vi "Read_Write_Calibrations.vi"(6 "Silent?":bool, 7 "Task":enum16{"Save", "Read", "List"}(ring)=enum."Read", 9 "Calibration name":string="Default", 11 "Settings in":T1={"Name of test"="", "Date"=timestamp(0 s since 1904-01-01), "Location"="", "Template"="", "Soundcard"="", "resolution"=32, "Sampling rate"=48000, "Ch1 Gain "=25.0, "Ch2 Gain"=10.0, "Sample time (s)"=0.3, "Pre-trigger (s)"=0.01, "Hammer Threshold"=10.0, "Positions"=12, "Taps/Position"=5, "Set Names"="", "Freq resolution"=10.0, "Hammer cutoff"=0.0, "Mic cutoff"=0.0, "Double bounce "=0.0, "Hammer Cal"=10.0, "dB Offset"=0.0, "Accel Cal"=10.0, "Vibrometer Cal"=0.0, "Mic Cal"=0.0, "Output"=2, "Voltage Cal"=1.0, "Vibrometer Port"="ASRL27::INSTR", "Range"=4, "High Pass"=2, "Bandwidth"=4, "X Range"=[], "Y Range"=[], "dB Spread"=0.0, "Trigger"=0, "Ch_1"=25, "Ch_2"=25, "flip?"=FALSE, "60Hz"=FALSE, "Time offset"=0.0, "Piezo Cal"=1.0, "Default Notes"=""} {"Ch_2" min=1 step=1; "Ch_1" min=1 max=100 step=1; "Trigger" items=["Hammer (force)", "Self-tap", "Spacebar"]; "Bandwidth" items=["1 kHz"=1, "5 kHz"=5, "10 kHz"=10, "25 kHz"=25, "50 kHz"=50, "100 kHz"=100]; "High Pass" items=["Off", "13 Hz", "104 Hz"]; "Range" items=["10 mm/s"=1, "20 mm/s"=2, "50 mm/s"=5, "100 mm/s"=10, "200 mm/s"=20, "500 mm/s"=50, "1 m/s"=100, "2 m/s"=200]; "Output" items=["Accelerometer", "Speed (from acceleration)", "Microphone", "Vibrometer", "Piezo"]; "Voltage Cal" format="%#_13g"; "Ch2 Gain" format="%#_13g"; "Ch1 Gain" format="%#_13g"; "Double bounce" min=0.0; "Mic cutoff" min=0.0 format="%#_4g"; "Hammer cutoff" min=0.0 format="%#_4g"; "Freq resolution" min=0.0; "Pre-trigger (s)" format="%#_13g"; "Date" format="%<%H:%M\n%d/%m/%y>T"; "resolution" items=["16 bit"=16, "24 bit"=24, "32 bit"=32]; "Sampling rate" items=["22050 samp/s"=22050, "44100 samp/s"=44100, "48000 samp/s"=48000]}) -> (0 "file":string, 1 "Cal files":string[](array[string]), 3 "Settings out":T1={"Name of test"="", "Date"=timestamp(0 s since 1904-01-01), "Location"="", "Template"="", "Soundcard"="", "resolution"=32, "Sampling rate"=48000, "Ch1 Gain "=25.0, "Ch2 Gain"=10.0, "Sample time (s)"=0.3, "Pre-trigger (s)"=0.01, "Hammer Threshold"=10.0, "Positions"=12, "Taps/Position"=5, "Set Names"="", "Freq resolution"=10.0, "Hammer cutoff"=0.0, "Mic cutoff"=0.0, "Double bounce "=0.0, "Hammer Cal"=10.0, "dB Offset"=0.0, "Accel Cal"=10.0, "Vibrometer Cal"=0.0, "Mic Cal"=0.0, "Output"=2, "Voltage Cal"=1.0, "Vibrometer Port"="ASRL27::INSTR", "Range"=4, "High Pass"=2, "Bandwidth"=4, "X Range"=[], "Y Range"=[], "dB Spread"=0.0, "Trigger"=0, "Ch_1"=25, "Ch_2"=25, "flip?"=FALSE, "60Hz"=FALSE, "Time offset"=0.0, "Piezo Cal"=1.0, "Default Notes"=""} {"Ch_2" min=1 step=1; "Ch_1" min=1 max=100 step=1; "Trigger" items=["Hammer (force)", "Self-tap", "Spacebar"]; "Bandwidth" items=["1 kHz"=1, "5 kHz"=5, "10 kHz"=10, "25 kHz"=25, "50 kHz"=50, "100 kHz"=100]; "High Pass" items=["Off", "13 Hz", "104 Hz"]; "Range" items=["10 mm/s"=1, "20 mm/s"=2, "50 mm/s"=5, "100 mm/s"=10, "200 mm/s"=20, "500 mm/s"=50, "1 m/s"=100, "2 m/s"=200]; "Output" items=["Accelerometer", "Speed (from acceleration)", "Microphone", "Vibrometer", "Piezo"]; "Voltage Cal" format="%#_13g"; "Ch2 Gain" format="%#_13g"; "Ch1 Gain" format="%#_13g"; "Double bounce" min=0.0; "Mic cutoff" min=0.0 format="%#_4g"; "Hammer cutoff" min=0.0 format="%#_4g"; "Freq resolution" min=0.0; "Pre-trigger (s)" format="%#_13g"; "Date" format="%<%H:%M\n%d/%m/%y>T"; "resolution" items=["16 bit"=16, "24 bit"=24, "32 bit"=32]; "Sampling rate" items=["22050 samp/s"=22050, "44100 samp/s"=44100, "48000 samp/s"=48000]})   [LabVIEW 2022 SP3]
uses:
  PreferencesControl.ctl
panel:
  out "filenames":string[](array[string])
  out "Path to Calibrations":path
  out "error out":errorcluster
  in  "error in":errorcluster
  # "Hz"
  # "dB"
  # "dB"
  # "sec"
  # "sec"
  # "mV/Pa"
  # "mV/m/s2"
  # "mV/mm/s"
  # "V/N"
  # "sec"
  # "sec"
  # "mV/N"
  # "a.u."
  # "a.u."
  # "sec"
  # "Hz"
  # "dB"
  # "dB"
  # "sec"
  # "sec"
  # "mV/Pa"
  # "mV/m/s2"
  # "mV/mm/s"
  # "V/N"
  # "sec"
  # "sec"
  # "mV/N"
  # "a.u."
  # "a.u."
  # "sec"
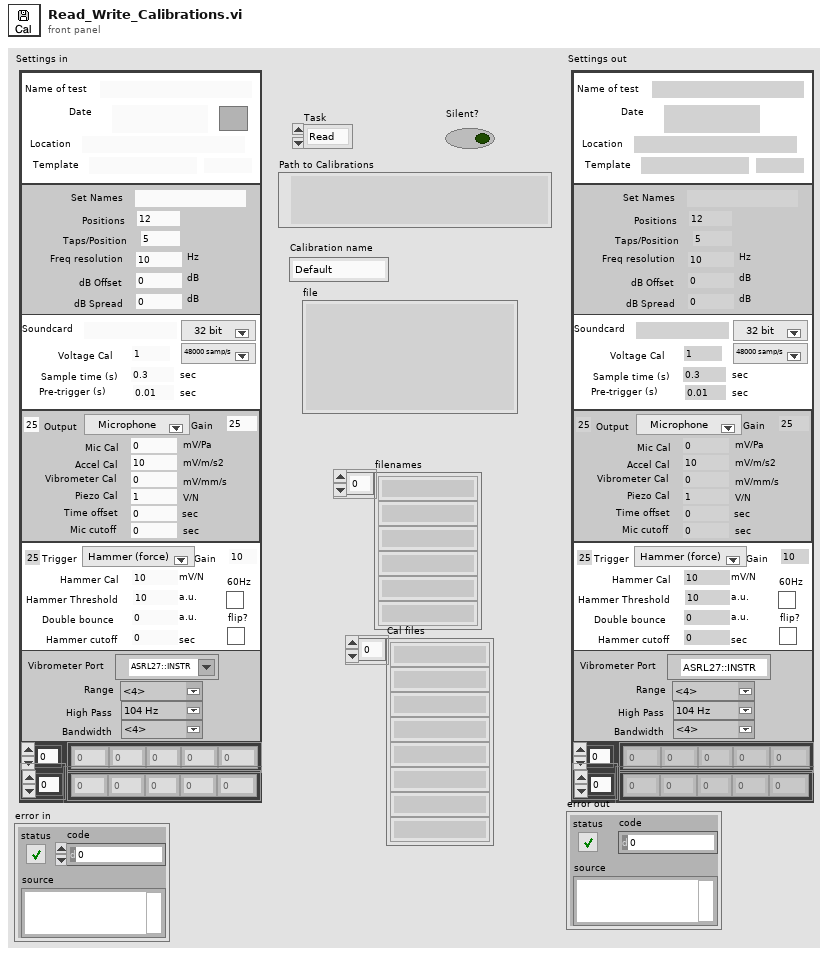
[diagram p1: front panel]
types:
  T1 = typedef "PreferencesControl.ctl" = cluster{"Name of test":string, "Date":timestamp, "Location":string, "Template":string, "Soundcard":string, "resolution":u16, "Sampling rate":u16, "Ch1 Gain ":dbl, "Ch2 Gain":dbl, "Sample time (s)":dbl, "Pre-trigger (s)":dbl, "Hammer Threshold":dbl, "Positions":i16, "Taps/Position":i16, "Set Names":string, "Freq resolution":dbl, "Hammer cutoff":dbl, "Mic cutoff":dbl, "Double bounce ":dbl, "Hammer Cal":dbl, "dB Offset":dbl, "Accel Cal":dbl, "Vibrometer Cal":dbl, "Mic Cal":dbl, "Output":u16, "Voltage Cal":dbl, "Vibrometer Port":refnum<visa-resource-name>, "Range":u16, "High Pass":u16, "Bandwidth":u16, "X Range":cluster{"Minimum":dbl, "Maximum":dbl, "Increment":dbl, "Minor Increment":dbl, "Start":dbl}[], "Y Range":cluster{"Minimum":dbl, "Maximum":dbl, "Increment":dbl, "Minor Increment":dbl, "Start":dbl}[], "dB Spread":dbl, "Trigger":u16, "Ch_1":u8, "Ch_2":u8, "flip?":bool, "60Hz":bool, "Time offset":dbl, "Piezo Cal":dbl, "Default Notes":string}
  T2 = cluster{"Voltage Cal":dbl, "Mic Cal":dbl, "Accel Cal":dbl, "Vibrometer Cal":dbl, "Hammer Cal":dbl, "Piezo Cal":dbl, "flip":dbl}
  T3 = cluster{"[0]":dbl, "[1]":dbl, "[2]":dbl, "[3]":dbl, "[4]":dbl, "[5]":dbl, "[6]":dbl}
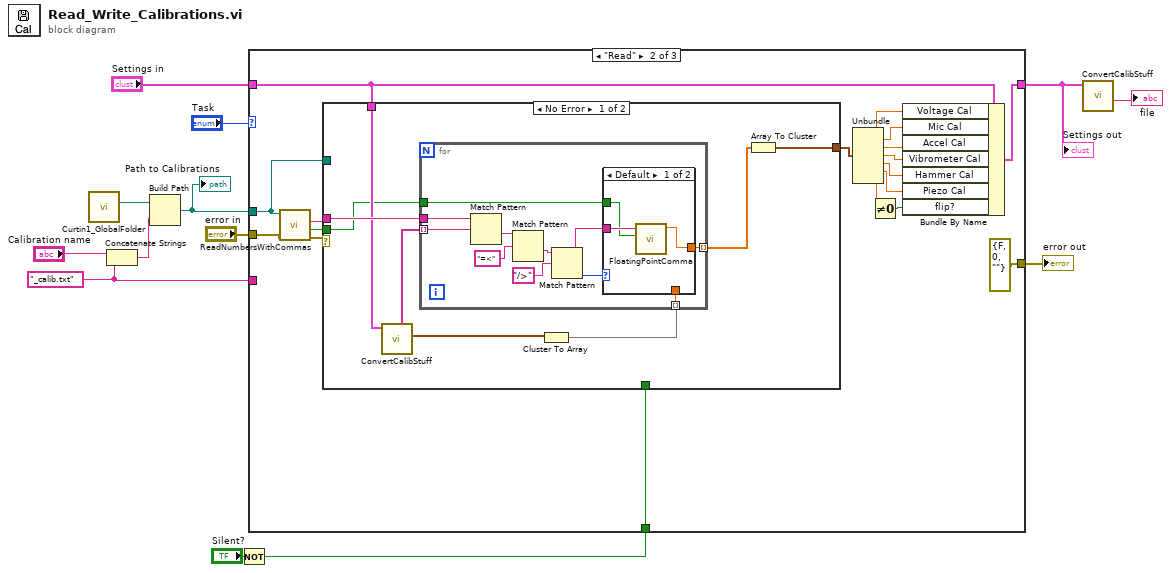
[diagram p0: block diagram]
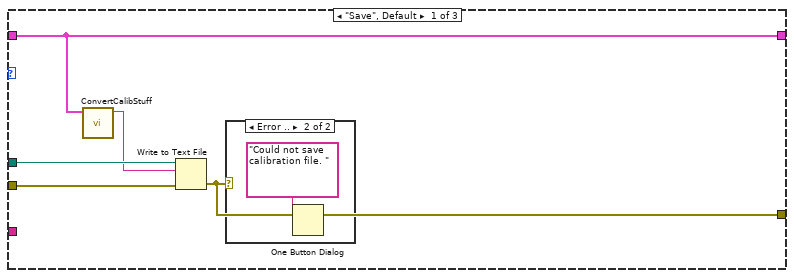
[diagram p2: hidden frame]
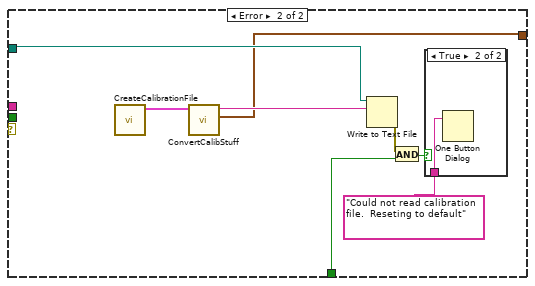
[diagram p5: hidden frame]
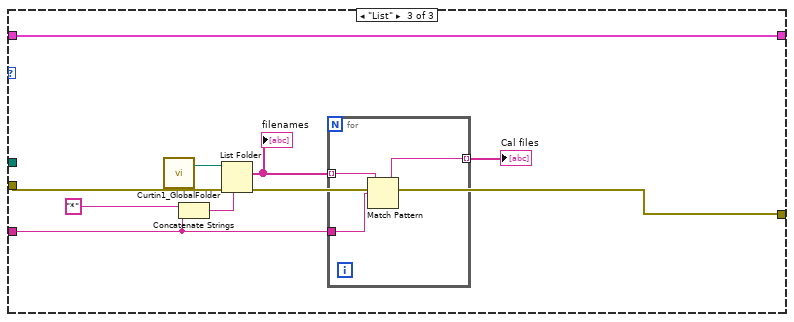
[diagram p7: hidden frame]
diagram:
  w5 = "_calib.txt" ("name or relative path")
  n1 = call "Curtin1_GlobalFolder.vi"() -> ("LabVIEW Data Path"=w13:path)  [unwired: 1 in, 1 out]
  n2 = Concatenate Strings("Calibration name", w5) -> (w6:string)
  n3 = Build Path(base path=w13, name or relative path=w6) -> (appended path=w12:path)
  "Path to Calibrations" <- w12
  n4 = Not(x="Silent?") -> (.not. x?=w3:bool)
  n5 = case shown="\"Read\"" "Task" {
    tunnel: w12 -> [w17 w25 _]
    tunnel: "error in" -> [w16 w24 w76]
    tunnel: "Settings in" -> [w18 w28 w78]
    tunnel: [w18 w31 w78] -> w2
    tunnel: [w14 errorcluster {"status"=FALSE, "code"=0, "source"=""} ("error out") w70] -> w8
    tunnel: w5 -> [_ _ w72]
    tunnel: w3 -> [_ w29 _]
    frame "Save", Default {
      n6 = call "ConvertCalibStuff.vi"("Settings in"=w18) -> ("File"=w15:string)  [unwired: 7 in, 3 out]
      n7 = Write to Text File(file (use dialog)=w17, text=w15, error in=w16) -> (error out=w14:errorcluster)  [unwired: 1 in, 2 out]
      n8 = case shown="Error .." w14 {
        frame No Error {
        }
        frame Error {
          n9 = One Button Dialog(message="Could not save calibration file. ") -> ()  [unwired: 1 in, 1 out]
        }
      }
    }
    frame "Read" {
      n10 = call "ReadNumbersWithCommas.vi"("error in"=w24, "file (use dialog)"=w25) -> ("error out"=w27:errorcluster, "comma?"=w23:bool, "text"=w26:string)  [unwired: 6 in, 1 out]
      n11 = case shown="No Error" w27 {
        tunnel: w26 -> [w45 _]
        tunnel: [w43 w61] -> w37
        tunnel: w25 -> [_ w68]
        tunnel: w29 -> [_ w65]
        tunnel: w28 -> [w41 _]
        tunnel: w23 -> [w38 _]
        frame No Error {
          n12 = call "ConvertCalibStuff.vi"("Settings in"=w41) -> ("cluster"=w40:T2, "titles"=w39:string[])  [unwired: 7 in, 2 out]
          n13 = Cluster To Array(cluster=w40) -> (array=w42:dbl[])
          n14 = for {
            tunnel: w45 -> [w52]
            tunnel: [w49] -> w44 mode=indexing
            tunnel: w42 -> [w48] mode=indexing
            tunnel: w39 -> [w47] mode=indexing
            tunnel: w38 -> [w46]
            n15 = Match Pattern(string=w52, regular expression=w47) -> (after substring=w53:string)  [unwired: 1 in, 3 out]
            n16 = Match Pattern(string=w53, regular expression="=<" ("format string")) -> (after substring=w54:string)  [unwired: 1 in, 3 out]
            n17 = Match Pattern(string=w54, regular expression="/>" ("format string")) -> (before substring=w50:string, offset past match=w51:i32)  [unwired: 1 in, 2 out]
            n18 = case shown="Default" w51 {
              tunnel: w50 -> [w59 _]
              tunnel: [w58 w60] -> w49
              tunnel: w48 -> [_ w60]
              tunnel: w46 -> [w57 _]
              frame Default {
                n19 = call "FloatingPointComma.vi"("Comma?"=w57, "String In"=w59) -> ("Numeric"=w58:dbl)  [unwired: 8 in, 1 out]
              }
              frame -1 {
              }
            }
          }
          n20 = Array To Cluster(array=w44) -> (cluster=w43:T3)
        }
        frame Error {
          n21 = call "CreateCalibrationFile.vi"() -> ("Settings out"=w63:T1)  [unwired: 11 in]
          n22 = call "ConvertCalibStuff.vi"("Settings in"=w63) -> ("cluster"=w61:T2, "File"=w62:string)  [unwired: 7 in, 2 out]
          n23 = Write to Text File(file (use dialog)=w68, text=w62) -> (error out=w66:errorcluster)  [unwired: 2 in, 2 out]
          n24 = And(x=w66, y=w65) -> (x .and. y?=w64:bool)
          n25 = case shown="True" w64 {
            tunnel: "Could not read calibration file.  Reseting to default" ("message") -> [_ w69]
            frame False {
            }
            frame True {
              n26 = One Button Dialog(message=w69) -> ()  [unwired: 1 in, 1 out]
            }
          }
        }
      }
      n27 = Unbundle(w37) -> ("Voltage Cal"=w36:dbl, "Mic Cal"=w35:dbl, "Accel Cal"=w34:dbl, "Vibrometer Cal"=w33:dbl, "Hammer Cal"=w32:dbl, "Piezo Cal"=w22:dbl, "flip"=w20:dbl)
      n28 = Not Equal To 0?(x=w20) -> (x != 0?=w21:bool)
      n29 = Bundle By Name(cluster=w28, "Voltage Cal"=w36, "Mic Cal"=w35, "Accel Cal"=w34, "Vibrometer Cal"=w33, "Hammer Cal"=w32, "Piezo Cal"=w22, "flip?"=w21) -> (w31:T1)
    }
    frame "List" {
      n30 = call "Curtin1_GlobalFolder.vi"() -> ("LabVIEW Data Path"=w77:path)  [unwired: 1 in, 1 out]
      n31 = Concatenate Strings("*" ("string"), w72) -> (w74:string)
      n32 = List Folder(path=w77, pattern=w74, error in=w76) -> (filenames=w73:string[], error out=w70:errorcluster)  [unwired: 1 in, 2 out]
      "filenames" <- w73
      n33 = for {
        tunnel: w73 -> [w81] mode=indexing
        tunnel: w72 -> [w80]
        tunnel: [w79] -> w71 mode=indexing
        n34 = Match Pattern(string=w81, regular expression=w80) -> (before substring=w79:string)  [unwired: 1 in, 3 out]
      }
      "Cal files" <- w71
    }
  }
  "Settings out" <- w2
  "error out" <- w8
  n35 = call "ConvertCalibStuff.vi"("Settings in"=w2) -> ("Text"=→"file":string)  [unwired: 7 in, 3 out]
